vi "Lian_Scavenger_Hunt.vi"() -> ()   [LabVIEW 2020]
uses:
  <vilib>/measure/NI_MABase.lvlib
  <vilib>/Analysis/NI_AALPro.lvlib
  <vilib>/Analysis/NI_AALBase.lvlib
  <vilib>/DAQmx/create/channels.llb/DAQmx Create Channel (AI-Voltage-Basic).vi
panel:
  in  "Cluster 3":cluster{}
  in  "Ring":u16(ring)
  in  "Cluster":cluster{}
  out "String":string
  in  "Dial":dbl(knob) scale=0.0..10.0
  out "Waveform Chart":dbl(graph)
  in  "Boolean":bool
  in  "Slide":dbl(slide) scale=0.0..10.0
  in  "Stop":bool
  in  "Numeric":dbl
  # "Indicators"
  # "Controls"
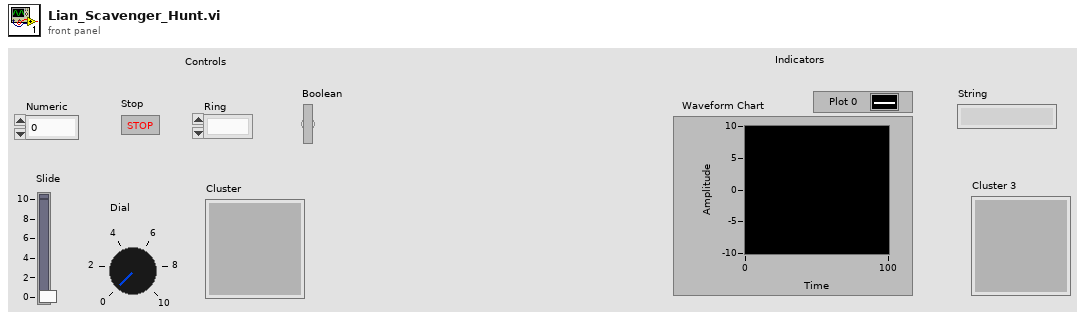
[diagram p1: front panel]
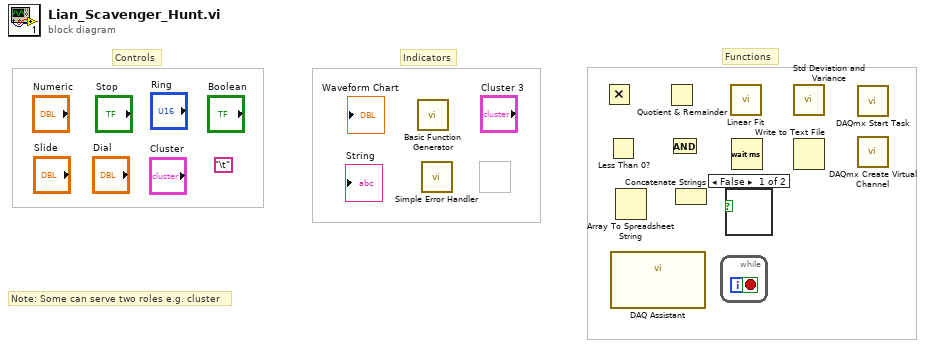
[diagram p0: block diagram]
diagram:
  (unwired) "\t"
  # "Note: Some can serve two roles e.g. cluster"
  # "Functions"
  # "Indicators"
  # "Controls"
  n1 = call <vilib>:"Basic Function Generator.vi"() -> ()  [unwired: 9 in, 3 out]
  n2 = call <vilib>:"Simple Error Handler.vi"() -> ()  [unwired: 5 in, 5 out]
  n3 = Multiply() -> ()  [unwired: 2 in, 1 out]
  n4 = Less Than 0?() -> ()  [unwired: 1 in, 1 out]
  n5 = call "DAQ Assistant"() -> ()  [unwired: 12 in]
  n6 = Array To Spreadsheet String() -> ()  [unwired: 3 in, 1 out]
  n7 = Quotient & Remainder() -> ()  [unwired: 2 in, 2 out]
  n8 = And() -> ()  [unwired: 2 in, 1 out]
  n9 = Concatenate Strings() -> ()  [unwired: 2 in, 1 out]
  n10 = while {
    stop <- _ stop-if-true
  }
  n11 = case shown="False" {
    selector: _ -> [_ _]
    frame False {
    }
    frame True {
    }
  }
  n12 = call <vilib>:"Linear Fit.vi"() -> ()  [unwired: 11 in, 5 out]
  n13 = Wait (ms)() -> ()  [unwired: 1 in, 1 out]
  n14 = call <vilib>:"Std Deviation and Variance.vi"() -> ()  [unwired: 2 in, 3 out]
  n15 = Write to Text File() -> ()  [unwired: 4 in, 3 out]
  n16 = call <vilib>:"DAQmx Start Task.vi"() -> ()  [unwired: 14 in, 2 out]
  n17 = call-poly <vilib>:"DAQmx Create Virtual Channel.vi"() -> ()  [unwired: 14 in, 2 out]
